vi "confirmation_input.vi"(7 "caller":refnum<vi>, 8 "error in (no error)":errorcluster, 11 "configuration":T1={"dialog_text"="", "boolean_text_1"="", "boolean_text_2"="", "boolean_text_3"="", "inner_color"=16711680, "outer_color"=6618880, "wait_s"=nan, "error_status"=FALSE, "error_source"="", "error_details"="", "string []"=[], "custom_entry"=FALSE}) -> (0 "error out":errorcluster, 3 "dialog_selection":T2)   [LabVIEW 2015, in "lv-dialog-interfaces.lvlib"]
uses:
  lv-dialog-interfaces.lvlib
  lv-dialog/api/v1/public/_controls/dialog_selection.ctl
  lv-dialog/api/v1/public/_controls/configuration.ctl
  _controls/dialog_type.ctl
  _controls/hmi_references.ctl
  <vilib>/event_ctls.llb/eventvkey.ctl
  lv-dialog/api/v1/v1.lvlib
panel:
  out "confirmation_dialog":string
  in  "confirmation_input":string
  in  "button 1":bool
  in  "button_2":bool
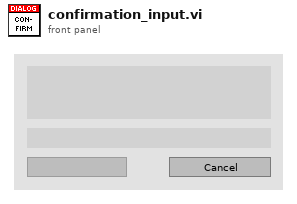
[diagram p1: front panel]
types:
  T1 = typedef "lv-dialog.lvlib/v1.lvlib/configuration.ctl" = cluster{"dialog_text":string, "boolean_text_1":string, "boolean_text_2":string, "boolean_text_3":string, "inner_color":u32, "outer_color":u32, "wait_s":dbl, "error_status":bool, "error_source":string, "error_details":string, "string []":string[], "custom_entry":bool}
  T2 = typedef "lv-dialog.lvlib/v1.lvlib/dialog_selection.ctl" = enum16{"null", "panel_closed", "button_1", "button_2", "button_3", "cancelled"}
  T3 = typedef "lv-dialog-interfaces.lvlib/dialog_type.ctl" = enum16{"null", "one_button", "two_button", "three_button", "confirmation", "busy_wait", "error", "busy_wait_embed", "combo_box", "data_entry_string", "data_entry_numeric"}
  T4 = typedef "lv-dialog-interfaces.lvlib/hmi_references.ctl" = cluster{"vi_reference":refnum<vi>, "caller":refnum<vi>, "dialog":refnum<vi>, "button_1":refnum<vi>, "button_2":refnum<vi>, "button_3":refnum<vi>, "busy":refnum<vi>, "error_glyph":refnum<vi>, "error_source":refnum<vi>, "error_text":refnum<vi>, "combo_box":refnum<vi>}
  T5 = typedef "eventvkey.ctl" = enum16{"ASCII", "Enter", "Return", "Shift", "Ctrl", "Alt", "Cmd", "Opt", "Caps", "NumLock", "Clear", "Break", "Up", "Down", "Left", "Right", "Insert", "Delete", "Home", "End", "PageUp", "PageDown", "Escape", "Help", "Pause", "ScrollLock", "F1", "F2", "F3", "F4", "F5", "F6", "F7", "F8", "F9", "F10", "F11", "F12", "F13", "F14", "F15", "F16", "F17", "F18", "F19", "F20", "F21", "F22", "F23", "F24", "Play", "VolumeUp", "VolumeDown", "Mute", "Two Byte Char"}
  T6 = enum8{"Enabled", "Disabled", "Disabled and Grayed Out"}
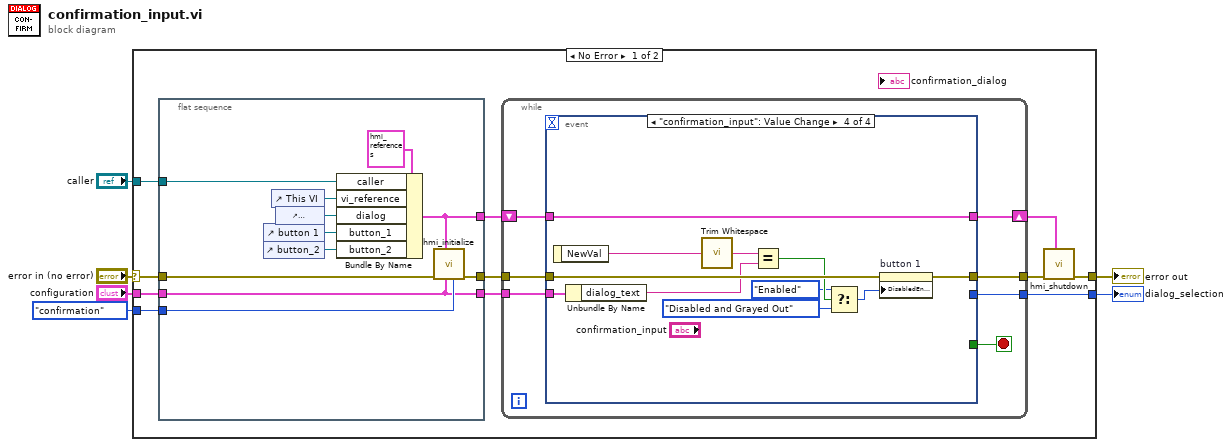
[diagram p0: block diagram]
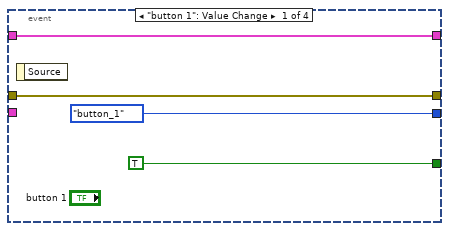
[diagram p2: hidden frame]
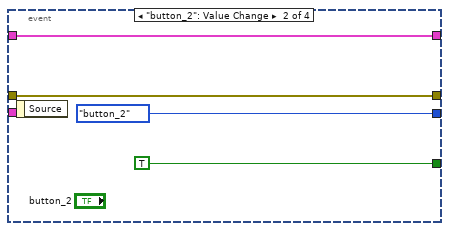
[diagram p3: hidden frame]
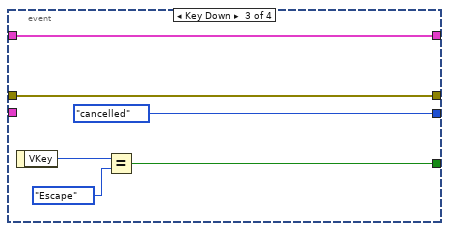
[diagram p4: hidden frame]
diagram:
  n1 = case shown="No Error" "error in (no error)" {
    selector: "error in (no error)" -> [w15 w61]
    tunnel: [w16 w61] -> w6
    tunnel: [w14 _] -> w4
    tunnel: "caller" -> [w13 _]
    tunnel: "configuration" -> [w12 _]
    tunnel: dialog_type."confirmation" ("dialog_type") -> [w11 _]
    frame No Error {
      n2 = flat-sequence {
        tunnel: w15 -> [w21]
        tunnel: w12 -> [w18]
        tunnel: [w22] -> w10
        tunnel: [w18] -> w9
        tunnel: w13 -> [w26]
        tunnel: w11 -> [w20]
        tunnel: [w19] -> w8
        frame #0 {
          n3 = control-ref of="button 1"() -> (w25:refnum<vi>)
          n4 = control-ref of="button_2"() -> (w24:refnum<vi>)
          n5 = control-ref of="This VI"() -> (w27:refnum<vi>)
          n6 = control-ref of="confirmation_dialog"() -> (w23:refnum<vi>)
          n7 = Bundle By Name(cluster=T4 {"vi_reference"=refnum, "caller"=refnum, "dialog"=refnum, "button_1"=refnum, "button_2"=refnum, "button_3"=refnum, "busy"=refnum, "error_glyph"=refnum, "error_source"=refnum, "error_text"=refnum, "combo_box"=refnum} ("references"), "caller"=w26, "vi_reference"=w27, "dialog"=w23, "button_1"=w25, "button_2"=w24) -> (w19:T4)
          n8 = call "hmi_initialize.vi"("dialog_type"=w20, "configuration"=w18, "references"=w19, "error in (no error)"=w21) -> ("error out"=w22:errorcluster)  [unwired: 7 in]
        }
      }
      n9 = while {
        tunnel: w10 -> [w32]
        tunnel: [w35] -> w14
        tunnel: w9 -> [w33]
        tunnel: [w31] -> w17
        shift-right: [w29] -> w7
        shift-left: w8 -> [w30]
        stop <- w34 stop-if-true
        n10 = event shown="[3] \"confirmation_input\": Value Change" {
          selector: _ -> [_ _ _ _]
          dyn-events: _ -> [_ _ _ _]
          timeout: _ -> [_ _ _ _]
          tunnel: [dialog_selection."button_1" ("dialog_selection") dialog_selection."button_2" ("dialog_selection") dialog_selection."cancelled" ("dialog_selection") _] -> w35
          tunnel: [TRUE TRUE w46 _] -> w34
          tunnel: w33 -> [_ _ _ w50]
          tunnel: w32 -> [w38 w41 w48 w59]
          tunnel: [w38 w41 w48 w57] -> w31
          tunnel: w30 -> [w36 w40 w47 w52]
          tunnel: [w36 w40 w47 w52] -> w29
          event "button 1": Value Change {
            n11 = event-data() -> ()  [unwired: 1 in, 1 out]
          }
          event "button_2": Value Change {
            n12 = event-data() -> ()  [unwired: 1 in, 1 out]
          }
          event Key Down {
            n13 = event-data() -> ("VKey"=w45:T5)  [unwired: 1 in]
            n14 = Equal?(x=w45, y=eventvkey."Escape" ("VKey")) -> (x = y?=w46:bool)
          }
          event "confirmation_input": Value Change {
            n15 = event-data() -> ("NewVal"=w58:string)  [unwired: 1 in]
            n16 = Unbundle By Name(w50) -> ("dialog_text"=w51:string)
            n17 = call <vilib>:"Trim Whitespace.vi"("string"=w58) -> ("trimmed string"=w60:string)  [unwired: 1 in]
            n18 = Equal?(x=w60, y=w51) -> (x = y?=w55:bool)
            n19 = Select(t=T6."Enabled" ("Disabled"), s=w55, f=T6."Disabled and Grayed Out" ("Disabled")) -> (s? t:f=w56:T6)
            n20 = property on="button 1" class="Bool"(error in=w59, "DisabledEnum"=w56) -> (error out=w57:errorcluster)  [unwired: 1 in, 1 out]
          }
        }
      }
      n21 = call "hmi_shutdown.vi"("references"=w7, "error in (no error)"=w17) -> ("error out"=w16:errorcluster)  [unwired: 9 in]
    }
    frame Error {
    }
  }
  "error out" <- w6
  "dialog_selection" <- w4
